vi "get table and column names.vi"() -> ()   [LabVIEW 2020]
uses:
  ADODB.lvclass
panel:
  in  "Database *.udl file":path=path "C:/Users/User/Desktop/Raman Program/Test Data/testDB.udl"
  out "Table and Column Info":T1(array[cluster])
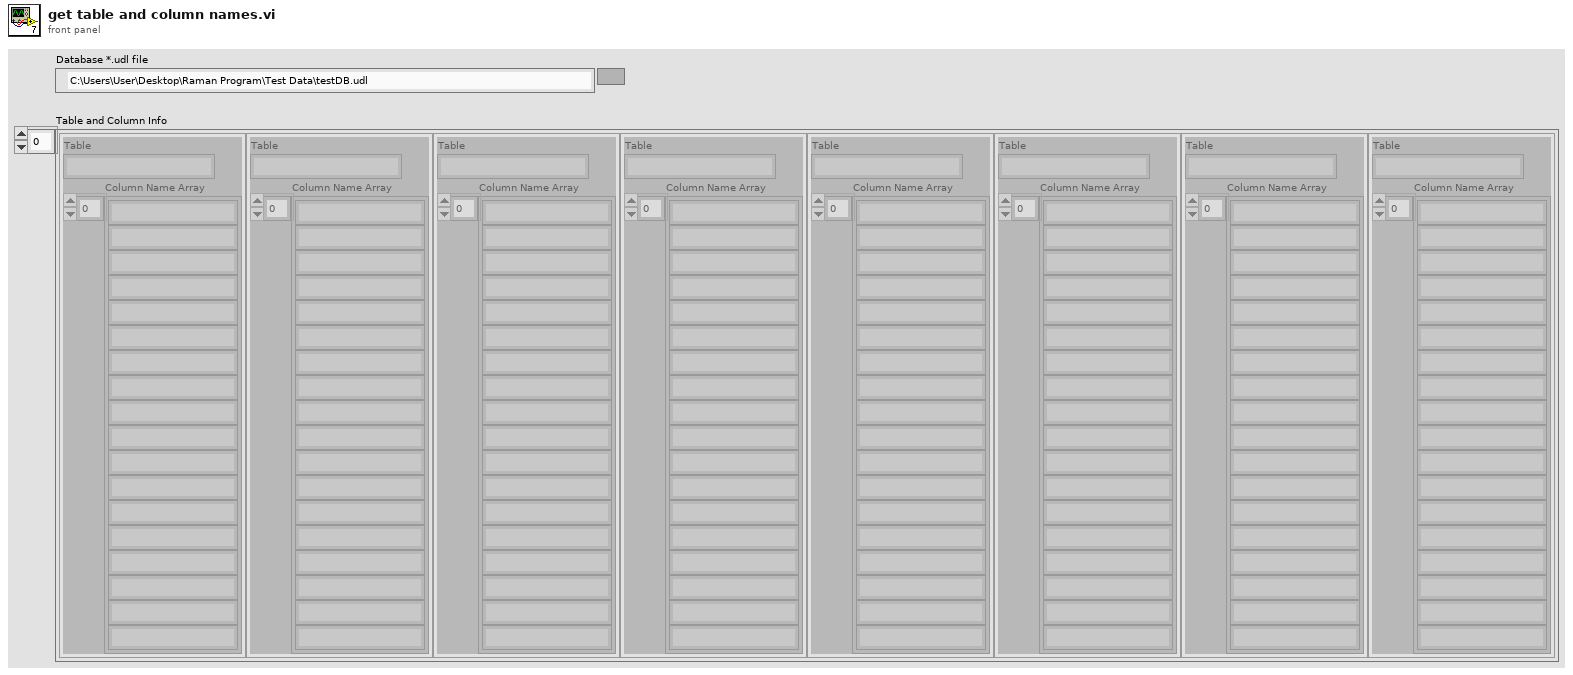
[diagram p1: front panel]
types:
  T1 = cluster{"Table":string, "Column Name Array":string[]}[]
  T2 = cluster{"Table":string, "Column Name Array":string[]}
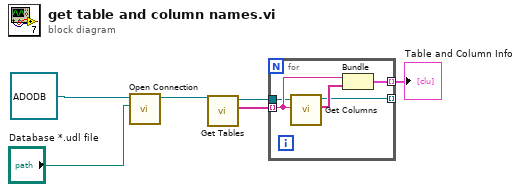
[diagram p0: block diagram]
diagram:
  n1 = call-dynamic "Open Connection.vi"("Connection Info (Member Data/Prompt)"="Database *.udl file", "ODBC in"=refnum<class "ADODB.lvclass"> refnum ("ADODB.lvclass")) -> ("ODBC out"=w5:refnum<class "ADODB.lvclass">)  [unwired: 8 in, 1 out]
  n2 = call-dynamic "Get Tables.vi"("ODBC in"=w5) -> ("Table Names"=w6:string[], "ODBC out"=w4:refnum<class "ADODB.lvclass">)  [unwired: 8 in, 1 out]
  n3 = for {
    tunnel: w6 -> [w10] mode=indexing
    tunnel: [w9] -> w3 mode=indexing
    tunnel: w4 -> [w8]
    tunnel: [w7] -> _ mode=indexing
    n4 = call-dynamic "Get Columns.vi"("Table Name"=w10, "ODBC in"=w8) -> ("Column Name Array"=w11:string[], "ODBC out"=w7:refnum<class "ADODB.lvclass">)  [unwired: 7 in, 1 out]
    n5 = Bundle("Table"=w10, "Column Name Array"=w11) -> (w9:T2)  [unwired: 1 in]
  }
  "Table and Column Info" <- w3
